vi "Get 2D U64.vi"(7 "key description":string, 8 "sections":string[](array[string]), 9 "numeric":u64[][](array[numeric]), 11 "info data":string) -> (0 "sections out":string[](array[string]), 1 "key found?":bool, 2 "value":u64[][](array[numeric]), 3 "info data out":string)   [LabVIEW 2020, in "infolib.lvlib"]
doc: "Reads matrix of unsigned 64 bit integers. If section is entered it searches the key in the section(s).\nInput 'numeric' can be used to set default value.\nIf key is not found, the output value is equal to 'numeric' input.\nIf key is found, and element of matrix cannot be converted into data type, the default value of output matrix element is based on:\n- first element of 'numeric' input if available\n- otherwise maximum of U64 is used."
uses:
  infolib.lvlib
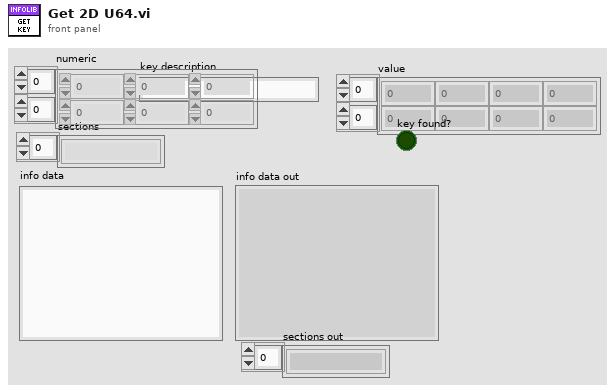
[diagram p1: front panel]
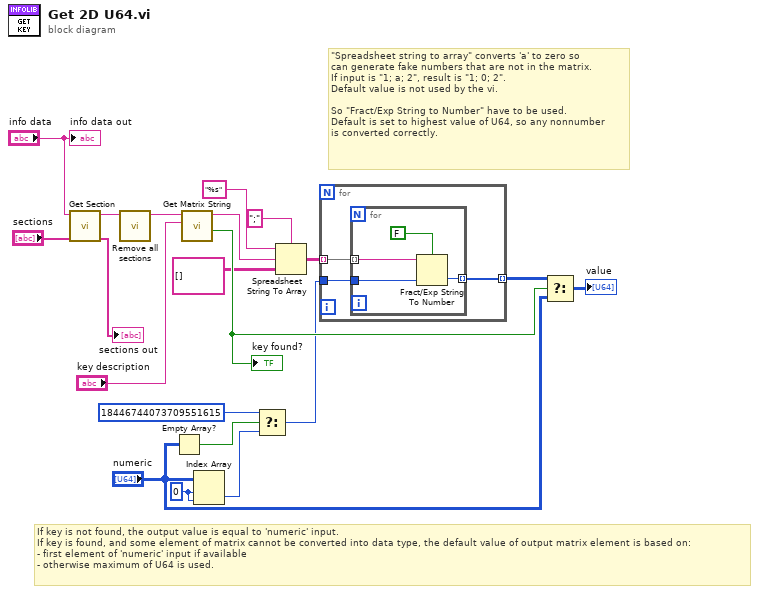
[diagram p0: block diagram]
diagram:
  w2 = 0 ("index (row)")
  # "If key is not found, the output value is equal to 'numeric' input.\nIf key is found, and some element of matrix cannot be converted into data type, the default value of output matrix element is based on:\n- first element of 'numeric' input if available\n- otherwise maximum of U64 is used."
  # "\"Spreadsheet string to array\" converts 'a' to zero so\ncan generate fake numbers that are not in the matrix.\nIf input is \"1; a; 2\", result is \"1; 0; 2\".\nDefault value is not used by the vi.\n\nSo \"Fract/Exp String to Number\" have to be used.\nDefault is set to highest value of U64, so any nonnumber\nis converted correctly."
  n1 = call "Get Section.vi"("sections"="sections", "info data"="info data") -> ("sections out"=→"sections out":string[], "section part"=w20:string)  [unwired: 7 in, 1 out]
  n2 = call "Remove all sections.vi"("info data"=w20) -> ("info data out"=w18:string)  [unwired: 10 in]
  n3 = Empty Array?(array="numeric") -> (empty?=w5:bool)
  n4 = call "Get Matrix String.vi"("matrix key"="key description", "info data"=w18) -> ("key found?"=w10:bool, "matrix part"=w16:string)  [unwired: 8 in]
  "key found?" <- w10
  n5 = Index Array(array="numeric", index (row)=w2, index (col)=w2) -> (element=w3:u64)
  n6 = Select(t=u64 18446744073709551615 ("default (0 DBL)"), s=w5, f=w3) -> (s? t:f=w1:u64)
  n7 = Spreadsheet String To Array(delimiter (Tab)=";", format string="%s" ("format string (%_20f)"), spreadsheet string=w16, array type (2D Dbl)=string[][] [] ("v")) -> (array=w8:string[][])
  n8 = for {
    tunnel: w8 -> [w23] mode=indexing
    tunnel: [w22] -> w7 mode=indexing
    tunnel: w1 -> [w21]
    n9 = for {
      tunnel: w23 -> [w26] mode=indexing
      tunnel: [w25] -> w22 mode=indexing
      tunnel: w21 -> [w24]
      n10 = Fract/Exp String To Number(use system decimal point (T)=FALSE, string=w26, default (0 dbl)=w24) -> (number=w25:u64)  [unwired: 1 in, 1 out]
    }
  }
  n11 = Select(t=w7, s=w10, f="numeric") -> (s? t:f=→"value":u64[][])
  "info data out" <- "info data"
